vi "Write Optimisation Strategy.vi"(8 "error in (no error)":errorcluster, 10 "Optimisation method":T1, 11 "Optimiser Cell in":refnum<class "Optimiser Cell.lvclass">) -> (0 "error out":errorcluster, 3 "Optimiser Cell out":refnum<class "Optimiser Cell.lvclass">)   [LabVIEW 2020, in "Run Utilities.lvlib" / "Optimiser Cell.lvclass"]
uses:
  Optimiser Cell.lvclass
  Optimisation Strategy.ctl
  Optimiser Cell.lvclass/Optimiser Cell.ctl
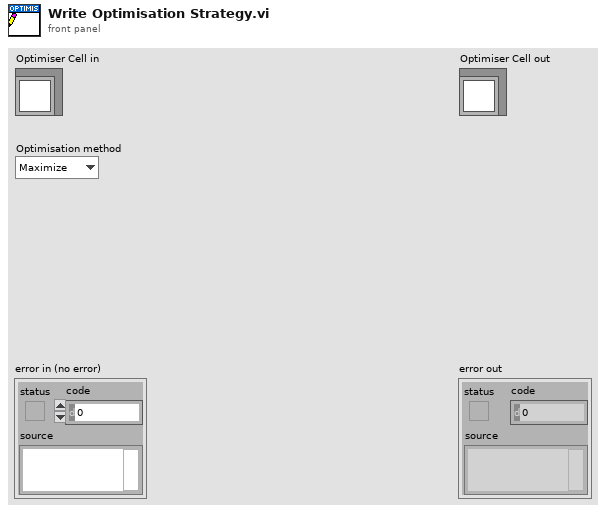
[diagram p1: front panel]
types:
  T1 = typedef "Run Utilities.lvlib/Optimiser Cell.lvclass/Optimisation Strategy.ctl" = enum16{"Maximize", "Minimize", "Value"}
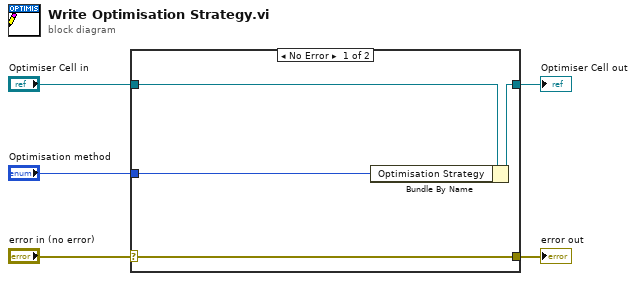
[diagram p0: block diagram]
diagram:
  n1 = case shown="No Error" "error in (no error)" {
    selector: "error in (no error)" -> [w9 w10]
    tunnel: [w9 w10] -> w4
    tunnel: [w7 w11] -> w2
    tunnel: "Optimiser Cell in" -> [w8 w11]
    tunnel: "Optimisation method" -> [w6 _]
    frame No Error {
      n2 = Bundle By Name(cluster=w8, "Optimisation Strategy"=w6) -> (w7:refnum<class "Optimiser Cell.lvclass">)
    }
    frame Error {
    }
  }
  "error out" <- w4
  "Optimiser Cell out" <- w2
